vi "Pcre2MatchContextCopy8.vi"(8 "error in":errorcluster, 11 "pMatchContext":u64 format="%.0x") -> (0 "error out":errorcluster, 2 "pCopyOfMatchContext":u64 format="%.0x", 3 "pMatchContext":u64 format="%.0x")   [LabVIEW 2021, in "libpcre2-8.lvlib"]
uses:
  libpcre2-8.lvlib
  libpcre2-8-x32.dll
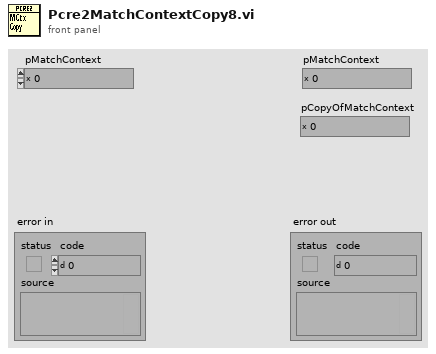
[diagram p1: front panel]
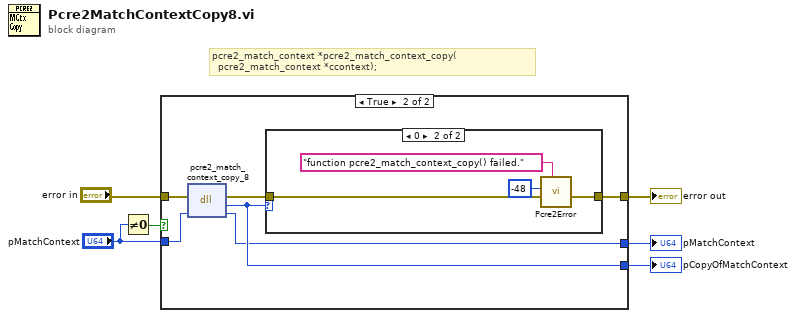
[diagram p0: block diagram]
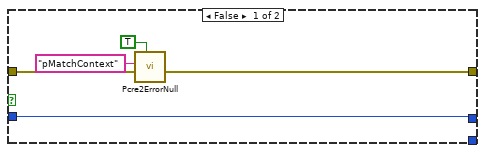
[diagram p2: hidden frame]
diagram:
  # "pcre2_match_context *pcre2_match_context_copy(\n  pcre2_match_context *ccontext);"
  n1 = Not Equal To 0?(x="pMatchContext") -> (x != 0?=w1:bool)
  n2 = case shown="True" w1 {
    tunnel: "error in" -> [w10 w17]
    tunnel: [w11 w15] -> w5
    tunnel: [_ w14] -> w4
    tunnel: "pMatchContext" -> [w7 w13]
    tunnel: [w7 w12] -> w2
    frame False {
      n3 = call "Pcre2ErrorNull.vi"("IsPointer? (F)"=TRUE, "error in"=w10, "What"="pMatchContext") -> ("error out"=w11:errorcluster)  [unwired: 8 in]
    }
    frame True {
      n4 = dll-call lib="libpcre2-8-x*.dll" fn="pcre2_match_context_copy_8"(error in=w17, "mcontext"=w13) -> (error out=w16:errorcluster, "CopyOfMatchContext"=w14:u64, "mcontext"=w12:u64)  [unwired: 2 in, 1 out]
      n5 = case shown="0" w14 {
        tunnel: w16 -> [w18 w21]
        tunnel: [w18 w20] -> w15
        frame Default {
        }
        frame 0 {
          n6 = call "Pcre2Error.vi"("message"="function pcre2_match_context_copy() failed.", "error in"=w21, "ErrorCode"=-48) -> ("error out"=w20:errorcluster)  [unwired: 8 in]
        }
      }
    }
  }
  "error out" <- w5
  "pCopyOfMatchContext" <- w4
  "pMatchContext" <- w2
